vi "4.vi"() -> ()   [LabVIEW 2020]
panel:
  out "result string":string
  in  "String":string
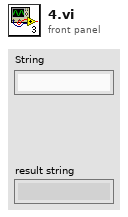
[diagram p1: front panel]
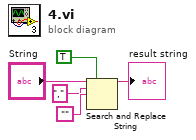
[diagram p0: block diagram]
diagram:
  n1 = Search and Replace String(replace all?=TRUE ("replace all? (F)"), input string="String", search string=",", replace string="") -> (result string=→"result string":string)  [unwired: 4 in, 3 out]
